vi "CSM - Global Log Error Handler.vi"(6 "Clear Error(T)":bool=TRUE, 7 "Place(\"\" to use VI's Name)":string, 8 "Error in":errorcluster caption="Error in (no error)") -> (0 "error out":errorcluster)   [LabVIEW 2020, in "Communicable State Machine.lvlib"]
doc: "<b>Inputs:</b>\n - <b>Error in</b>:\n - <b>From Who</b>:\n - <b>ModuleName</b>:\n - <b>Log</b>:\n - <b>Arguments</b>:\n\n<b>Outputs:</b>\n - <b>error out</b>:"
uses:
  Communicable State Machine.lvlib
  _CSM_GlobalLog_MSG_TYPE.ctl
  _CSM_GlobalLog_MSG.ctl
  _CSM_Response Source Message.ctl
  CSM - Make String Arguments Safe.vi
  CSM - Keywords.vi
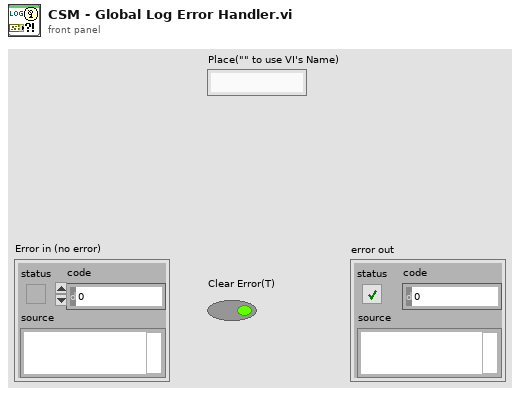
[diagram p1: front panel]
types:
  T1 = typedef "Communicable State Machine.lvlib/_CSM_GlobalLog_MSG_TYPE.ctl" = enum16{"User Log", "State Change", "Status", "Interrupt", "Register", "Unregister", "Error Log", "Module Created", "Module Destroyed"}
  T2 = typedef "Communicable State Machine.lvlib/_CSM_GlobalLog_MSG.ctl" = cluster{"Name(\"\" to use uuid)":string, "Current State":string, "Arguments":string, "Source Message":T3, "Source Module":string, "Complete(T)/Start(F)":bool, "LogType":T1}
  T3 = typedef "Communicable State Machine.lvlib/_CSM_Response Source Message.ctl" = cluster{"‘State":string, "’Arguments":string, "’Error":errorcluster}
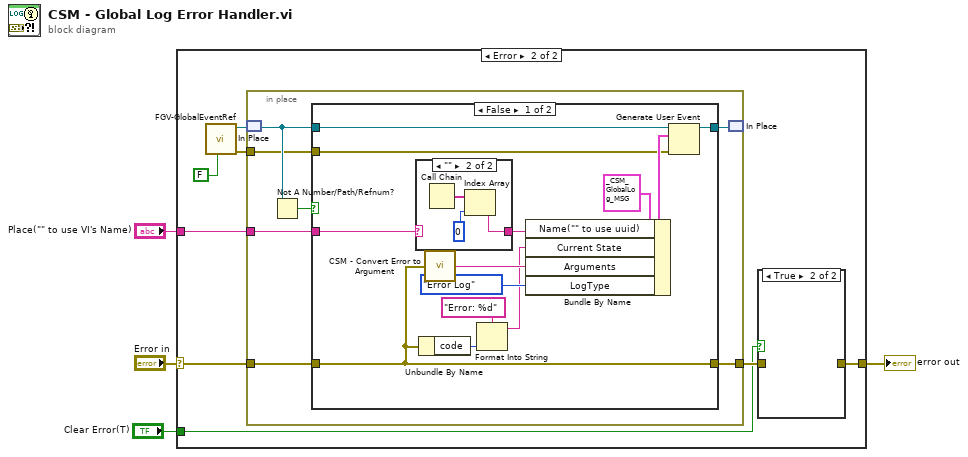
[diagram p0: block diagram]
diagram:
  n1 = case shown="Error" "Error in" {
    selector: "Error in" -> [w5 w12]
    tunnel: [w5 w10] -> w4
    tunnel: "Place(\"\" to use VI's Name)" -> [_ w13]
    tunnel: "Clear Error(T)" -> [_ w9]
    frame No Error {
    }
    frame Error {
      n2 = call "FGV-GlobalEventRef.vi"("Create(F)"=FALSE) -> ("error out"=w7:errorcluster, "CSM Global Log Event"=w8:refnum<user-event>)  [unwired: 9 in]
      n3 = in-place {
        in-place-border: w13 -> [w18]
        in-place-border: w7 -> [w17]
        in-place-border: w12 -> [w16]
        in-place-border: [w15] -> w11
        n4 = in-place-match #1(w8) -> (w20:refnum<user-event>)
        n5 = Not A Number/Path/Refnum?(number/path/refnum=w20) -> (NaN/Path/Refnum?=w21:bool)
        n6 = case shown="False" w21 {
          tunnel: w20 -> [w34 w40]
          tunnel: w18 -> [w24 _]
          tunnel: [w31 w40] -> w19
          tunnel: w17 -> [w28 _]
          tunnel: w16 -> [w22 w39]
          tunnel: [w22 w39] -> w15
          frame False {
            n7 = case shown="\"\"" w24 {
              selector: w24 -> [w35 _]
              tunnel: [w35 w36] -> w23
              frame Default {
              }
              frame "" {
                n8 = Call Chain() -> (call chain=w37:string[])
                n9 = Index Array(array=w37, index=0 ("Index")) -> (element=w36:string)
              }
            }
            n10 = Unbundle By Name(w22) -> ("code"=w27:i32)
            n11 = call "CSM - Convert Error to Argument.vi"("error in (no error)"=w22) -> ("Arguments"=w29:string)  [unwired: 4 in]
            n12 = Format Into String(format string="Error: %d", w27) -> (resulting string=w25:string)  [unwired: 2 in, 1 out]
            n13 = Bundle By Name(cluster=T2 {"Name(\"\" to use uuid)"="", "Current State"="", "Arguments"="", "Source Message"={"‘State"="", "’Arguments"="", "’Error"={"status"=FALSE, "code"=0, "source"=""}}, "Source Module"="", "Complete(T)/Start(F)"=FALSE, "LogType"=enum."User Log"} ("event data"), "Name(\"\" to use uuid)"=w23, "Current State"=w25, "Arguments"=w29, "LogType"=_CSM_GlobalLog_MSG_TYPE."Error Log" ("Type")) -> (w32:T2)
            n14 = Generate User Event(user event=w34, event data cluster=w32, error in=w28) -> (user event out=w31:refnum<user-event>)  [unwired: 1 in, 1 out]
          }
          frame True {
          }
        }
        n15 = in-place-match #1(w19) -> ()  [unwired: 1 out]
      }
      n16 = case shown="True" w9 {
        tunnel: w11 -> [w14 _]
        tunnel: [w14 _] -> w10
        frame False {
        }
        frame True {
        }
      }
    }
  }
  "error out" <- w4
